vi "LIGHT.vi"(1 "Disjoncteur general":bool, 2 "Disjonct":bool, 3 "Interrupteur":bool) -> (0 "LED":bool)   [LabVIEW 2024]
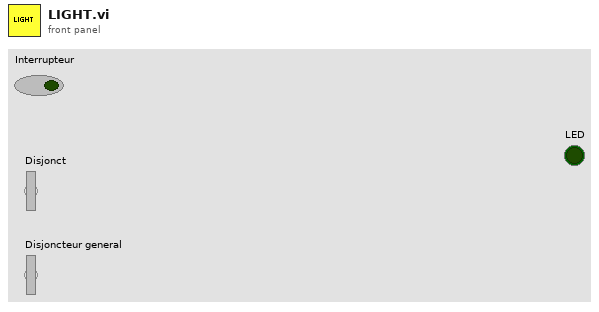
[diagram p1: front panel]
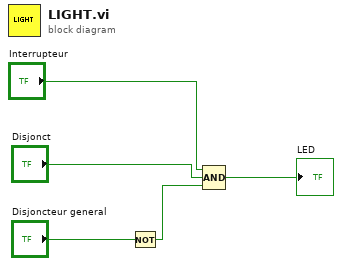
[diagram p0: block diagram]
diagram:
  n1 = Not(x="Disjoncteur general") -> (.not. x?=w5:bool)
  n2 = Compound Arithmetic op=AND ("Opérateur arithmétique")("Interrupteur", "Disjonct", w5) -> (→"LED":bool)
